vi "Set Cells in Existing File.vi"() -> ()   [LabVIEW 2013]
uses:
  Data/Polymorphic VIs/Set Cell (String).vi
  Data/Polymorphic VIs/Set Cell (DBL).vi
panel:
  in  "Worksheet":i32
  in  "File Name":path=path "C:/PhaeronGit/LVNPOI/Scratch/test.xls"
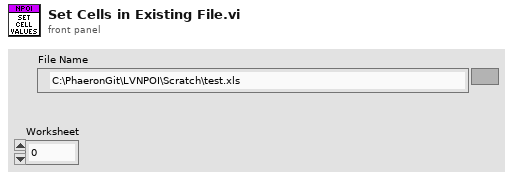
[diagram p1: front panel]
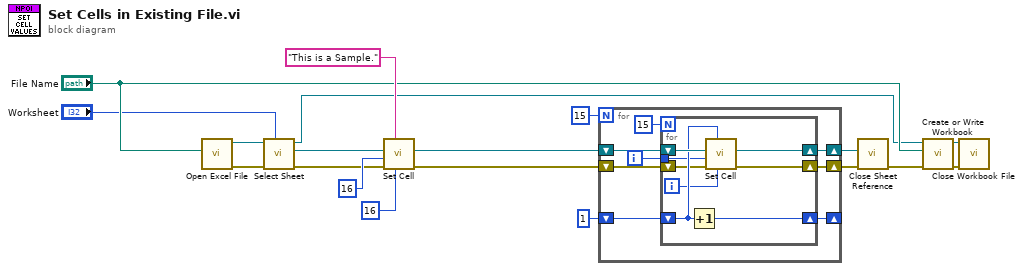
[diagram p0: block diagram]
diagram:
  n1 = call "Open Excel File.vi"("File Name"="File Name") -> ("error out"=w6:errorcluster, "IWorkbook Reference Out"=w5:refnum<k24>)  [unwired: 9 in]
  n2 = call "Select Sheet.vi"("Sheet (0)"="Worksheet", "error in (no error)"=w6, "IWorkbook Reference"=w5) -> ("error out"=w3:errorcluster, "Sheet Reference"=w1:refnum<k24>, "IWorkbook Reference"=w2:refnum<k24>)  [unwired: 6 in]
  n3 = call-poly "Set Cell.vi"("Column"=16 ("column"), "Value"="This is a Sample." ("value"), "error in (no error)"=w3, "Row"=16 ("rownum"), "Sheet Reference"=w1) -> ("error out"=w13:errorcluster, "Sheet Reference out"=w14:refnum<k24>)  [unwired: 5 in]
  n4 = for {
    N: 15 -> [_]
    shift-right: [w21] -> w9
    shift-left: w14 -> [w24]
    shift-right: [w20] -> w10
    shift-left: w13 -> [w22]
    shift-right: [w26] -> _
    shift-left: 1 -> [w27]
    i -> [w23]
    n5 = for {
      N: 15 -> [_]
      shift-right: [w35] -> w26
      shift-left: w27 -> [w33]
      shift-right: [w28] -> w20
      shift-left: w22 -> [w29]
      tunnel: w23 -> [w32]
      shift-right: [w30] -> w21
      shift-left: w24 -> [w34]
      i -> [w31]
      n6 = Increment(x=w33) -> (x+1=w35:i32)
      n7 = call-poly "Set Cell.vi"("Column"=w31, "Value"=w33, "error in (no error)"=w29, "Row"=w32, "Sheet Reference"=w34) -> ("error out"=w28:errorcluster, "Sheet Reference out"=w30:refnum<k24>)  [unwired: 5 in]
    }
  }
  n8 = call "Close Sheet Reference.vi"("error in (no error)"=w10, "Sheet Reference"=w9) -> ("error out"=w8:errorcluster)  [unwired: 9 in]
  n9 = call "Create or Write Workbook.vi"("error in (no error)"=w8, "File Name"="File Name", "IWorkbook Reference"=w2) -> ("error out"=w11:errorcluster, "IWorkbook Reference Out"=w12:refnum<k24>)  [unwired: 7 in]
  n10 = call "Close Workbook File.vi"("error in (no error)"=w11, "IWorkbook Reference"=w12) -> ()  [unwired: 9 in, 1 out]
